vi "倒计时器.vi"() -> ()   [LabVIEW 2017]
panel:
  out "倒计时":string
  in  "停止":bool
  out "布尔":bool
  in  "开始倒计时":bool
  in  "定时时间选择":enum16{"20秒", "10秒", "6秒"}(ring)
  # "倒 计 时 器"
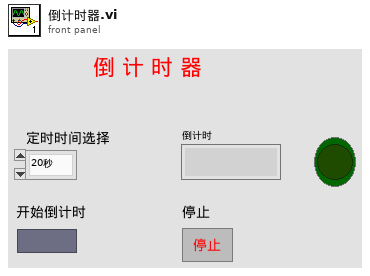
[diagram p1: front panel]
types:
  T1 = enum8{"Enabled", "Disabled", "Disabled and Grayed Out"}
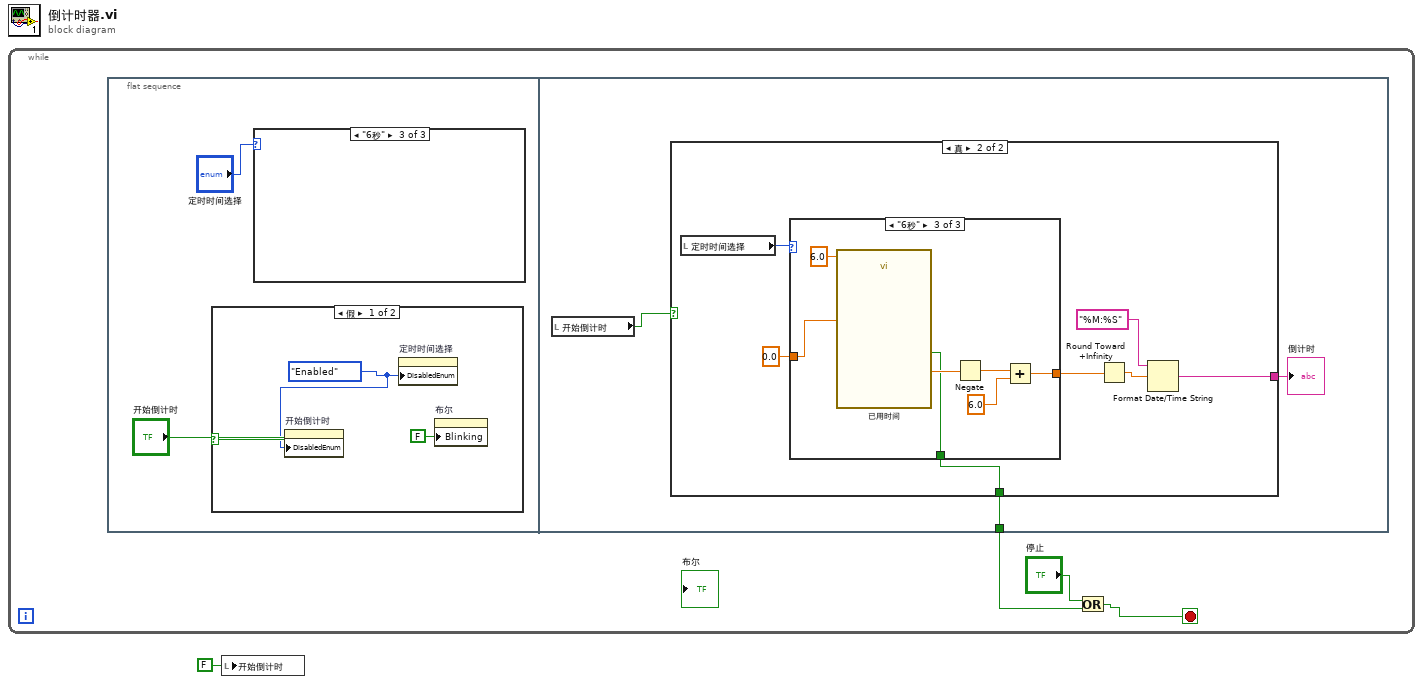
[diagram p0: block diagram]
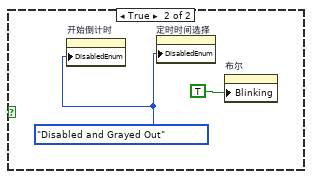
[diagram p2: hidden frame]
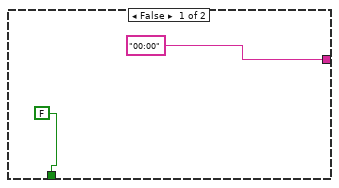
[diagram p5: hidden frame]
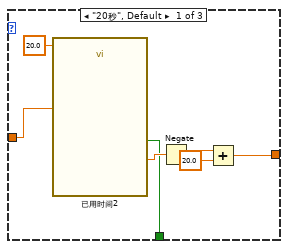
[diagram p6: hidden frame]
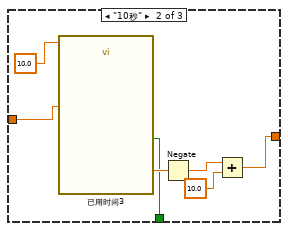
[diagram p7: hidden frame]
diagram:
  n1 = while {
    stop <- w2 stop-if-true
    n2 = flat-sequence {
      tunnel: [w13] -> w3
      frame #0 {
        n3 = case shown="假" "开始倒计时" {
          frame False {
            w7 = T1."Enabled" ("禁用")
            n4 = property on="开始倒计时" class="Bool (严格)"("DisabledEnum"=w7) -> ()  [unwired: 2 in, 2 out]
            n5 = property on="定时时间选择" class="Enum (严格)"("DisabledEnum"=w7) -> ()  [unwired: 2 in, 2 out]
            n6 = property on="布尔" class="Bool (严格)"("Blinking"=FALSE ("闪烁")) -> ()  [unwired: 2 in, 2 out]
          }
          frame True {
            w9 = T1."Disabled and Grayed Out" ("禁用")
            n7 = property on="开始倒计时" class="Bool (严格)"("DisabledEnum"=w9) -> ()  [unwired: 2 in, 2 out]
            n8 = property on="定时时间选择" class="Enum (严格)"("DisabledEnum"=w9) -> ()  [unwired: 2 in, 2 out]
            n9 = property on="布尔" class="Bool (严格)"("Blinking"=TRUE ("闪烁")) -> ()  [unwired: 2 in, 2 out]
          }
        }
        n10 = case shown="\"6秒\"" "定时时间选择" {
          frame "20秒", Default {
          }
          frame "10秒" {
          }
          frame "6秒" {
          }
        }
      }
      frame #1 {
        n11 = local read "开始倒计时"() -> (w12:bool)
        n12 = case shown="真" w12 {
          tunnel: [FALSE w20] -> w13
          tunnel: ["00:00" ("date/time string") w16] -> w11
          frame False {
          }
          frame True {
            n13 = local read "定时时间选择"() -> (w22:enum16{"20秒", "10秒", "6秒"})
            n14 = case shown="\"6秒\"" w22 {
              tunnel: [w25 w32 w39] -> w19
              tunnel: 0.0 ("Set Start Time (s)") -> [w24 w31 w38]
              tunnel: [w23 w30 w37] -> w20
              frame "20秒", Default {
                n15 = call "已用时间2"("Time Target (s)"=20.0, "Set Start Time (s)"=w24) -> ("Elapsed Time (s)"=w28:dbl, "Time has Elapsed"=w23:bool)  [unwired: 10 in, 6 out]
                n16 = Negate(x=w28) -> (-x=w27:dbl)
                n17 = Add(x=w27, y=20.0) -> (x+y=w25:dbl)
              }
              frame "10秒" {
                n18 = call "已用时间3"("Time Target (s)"=10.0, "Set Start Time (s)"=w31) -> ("Elapsed Time (s)"=w35:dbl, "Time has Elapsed"=w30:bool)  [unwired: 10 in, 6 out]
                n19 = Negate(x=w35) -> (-x=w34:dbl)
                n20 = Add(x=w34, y=10.0) -> (x+y=w32:dbl)
              }
              frame "6秒" {
                n21 = call "已用时间"("Time Target (s)"=6.0, "Set Start Time (s)"=w38) -> ("Elapsed Time (s)"=w42:dbl, "Time has Elapsed"=w37:bool)  [unwired: 10 in, 6 out]
                n22 = Negate(x=w42) -> (-x=w41:dbl)
                n23 = Add(x=w41, y=6.0) -> (x+y=w39:dbl)
              }
            }
            n24 = Round Toward +Infinity(x=w19) -> (ceil(x): smallest int >= x=w18:dbl)
            n25 = Format Date/Time String(time format string (%c)="%M:%S" ("时间格式字符串(%c)"), seconds (now)=w18) -> (date/time string=w16:string)  [unwired: 1 in]
          }
        }
        "倒计时" <- w11
      }
    }
    n26 = Or(x="停止", y=w3) -> (x .or. y?=w2:bool)
  }
  n27 = local write "开始倒计时"(FALSE ("开始倒计时")) -> ()
